vi "Filter vi.lib VIs.vi"(8 "Error In":errorcluster, 11 "VIs In":T1[](array[typedef])) -> (0 "Error Out":errorcluster, 3 "VIs Out":T1[](array[typedef]))   [LabVIEW 2018, in "Bookmark Manager.lvlib"]
uses:
  Bookmark Manager.lvlib
  Controls/VI Identifier.ctl
  <vilib>/addons/analyzer/_analyzerctrls.llb/VIAnCtl Analysis App Info.ctl
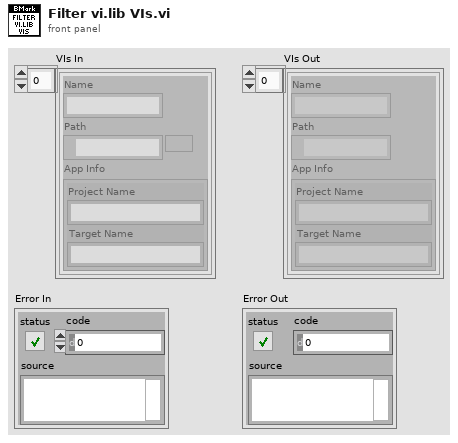
[diagram p1: front panel]
types:
  T1 = typedef "Bookmark Manager.lvlib/VI Identifier.ctl" = cluster{"Name":string, "Path":path, "App Info":T2}
  T2 = typedef "VIAnCtl Analysis App Info.ctl" = cluster{"Project Name":string, "Target Name":string}
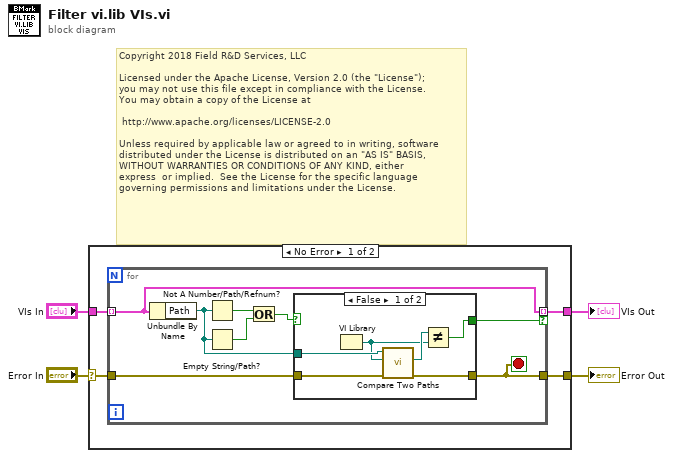
[diagram p0: block diagram]
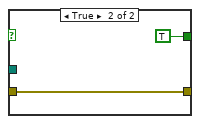
[diagram p2: hidden frame]
diagram:
  # "Copyright 2018 Field R&D Services, LLC\n\nLicensed under the Apache License, Version 2.0 (the \"License\");\nyou may not use this file except in compliance with the License.\nYou may obtain a copy of the License at\n\n\thttp://www.apache.org/licenses/LICENSE-2.0\n\nUnless required by applicable law or agreed to in writing, software\ndistributed under the License is distributed on an \"AS IS\" BASIS,\nWITHOUT WARRANTIES OR CONDITIONS OF ANY KIND, either \nexpress  or implied.  See the License for the specific language \ngoverning permissions and limitations under the License."
  n1 = case shown="No Error" "Error In" {
    selector: "Error In" -> [w5 w26]
    tunnel: [w8 w26] -> w4
    tunnel: "VIs In" -> [w7 w25]
    tunnel: [w6 w25] -> w1
    frame No Error {
      n2 = for {
        tunnel: w7 -> [w15] mode=indexing
        tunnel: w5 -> [w16]
        tunnel: [w13] -> w8
        tunnel: [w15] -> w6 mode=indexing if=w14
        stop <- w13 stop-if-true
        n3 = Unbundle By Name(w15) -> ("Path"=w10:path)
        n4 = Not A Number/Path/Refnum?(number/path/refnum=w10) -> (NaN/Path/Refnum?=w12:bool)
        n5 = Empty String/Path?(string/path=w10) -> (empty?=w11:bool)
        n6 = Or(x=w12, y=w11) -> (x .or. y?=w9:bool)
        n7 = case shown="False" w9 {
          tunnel: w10 -> [w22 _]
          tunnel: w16 -> [w21 w24]
          tunnel: [w20 w24] -> w13
          tunnel: [w17 TRUE] -> w14
          frame False {
            n8 = VI Library() -> (path=w18:path)
            n9 = call <vilib>:"Compare Two Paths.vi"("error in (no error)"=w21, "Path 2"=w18, "Path 1"=w22) -> ("error out"=w20:errorcluster, "Common Path"=w19:path)  [unwired: 5 in, 2 out]
            n10 = Not Equal?(x=w19, y=w18) -> (x != y?=w17:bool)
          }
          frame True {
          }
        }
      }
    }
    frame Error {
    }
  }
  "Error Out" <- w4
  "VIs Out" <- w1
